vi "Element Type.vi"(11 "DblPopupControl in":refnum<class "DblPopupControl.lvclass">) -> (2 "Element Type":string)   [LabVIEW 2020, in "VolatusGUIElements.lvlib" / "DblPopupControl.lvclass"]
uses:
  DblPopupControl.lvclass
  DblPopupControl.lvclass/DblPopupControl.ctl
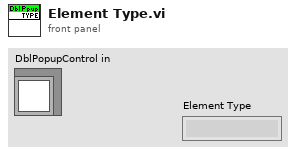
[diagram p1: front panel]
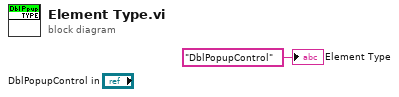
[diagram p0: block diagram]
diagram:
  "Element Type" <- "DblPopupControl" ("Element Type")
